vi "SEA_TORQUE_CONTROL_BENCHMARKING_TEST.vi"() -> ()   [LabVIEW 2019]
uses:
  <vilib>/FPGAPlugInAG/sbRIO-9627/niLvFpga_Open_sbRIO-9627.vi
  <vilib>/rvi/interface/common/dynamic/niFpgaDynamicAddResources.vi
  <vilib>/Utility/error.llb/Error Cluster From Error Code.vi
  <vilib>/rvi/errors/niLvFpgaAdjustHostInterfaceError.vi
  <vilib>/FPGAPlugInAG/Dynamic/niLvFpga_Close_Dynamic.vi
  <vilib>/rvi/interface/nirviOpenFPGA/nirviOpenFPGA.xnode
  FPGA Bitfiles/seafinalexperime_FPGATarget_SEALOWERLEVELCON_meT+vsors+U.lvbitx
  SEA_LOWER_LEVEL_CONTROL.vi
  <vilib>/rvi/interface/nirviReadWriteControl/nirviReadWriteControl.xnode
  <vilib>/rvi/interface/nirviCloseFPGA/nirviCloseFPGA.xnode
  NiFpgaLv.dll
  <vilib>/rvi/interface/Simulation/niFpgaSimulationCallBeginRW.vi
panel:
  out "Loop rate":u32
  in  "Position Reset":bool
  in  "Position Reset joint side":bool
  in  "KpGain":sgl
  out "Current":cluster{sgl, "Filtered Current(M2)":sgl}(graph)
  out "Torque":cluster{sgl, sgl}(graph)
  out "control_ip":sgl
  out "motor direction":bool
  in  "lower limit":sgl
  in  "upper limit":sgl
  in  "Kp":sgl
  in  "Amplitude":sgl
  in  "frequency":sgl
  in  "Current Offset":sgl
  in  "stop":bool
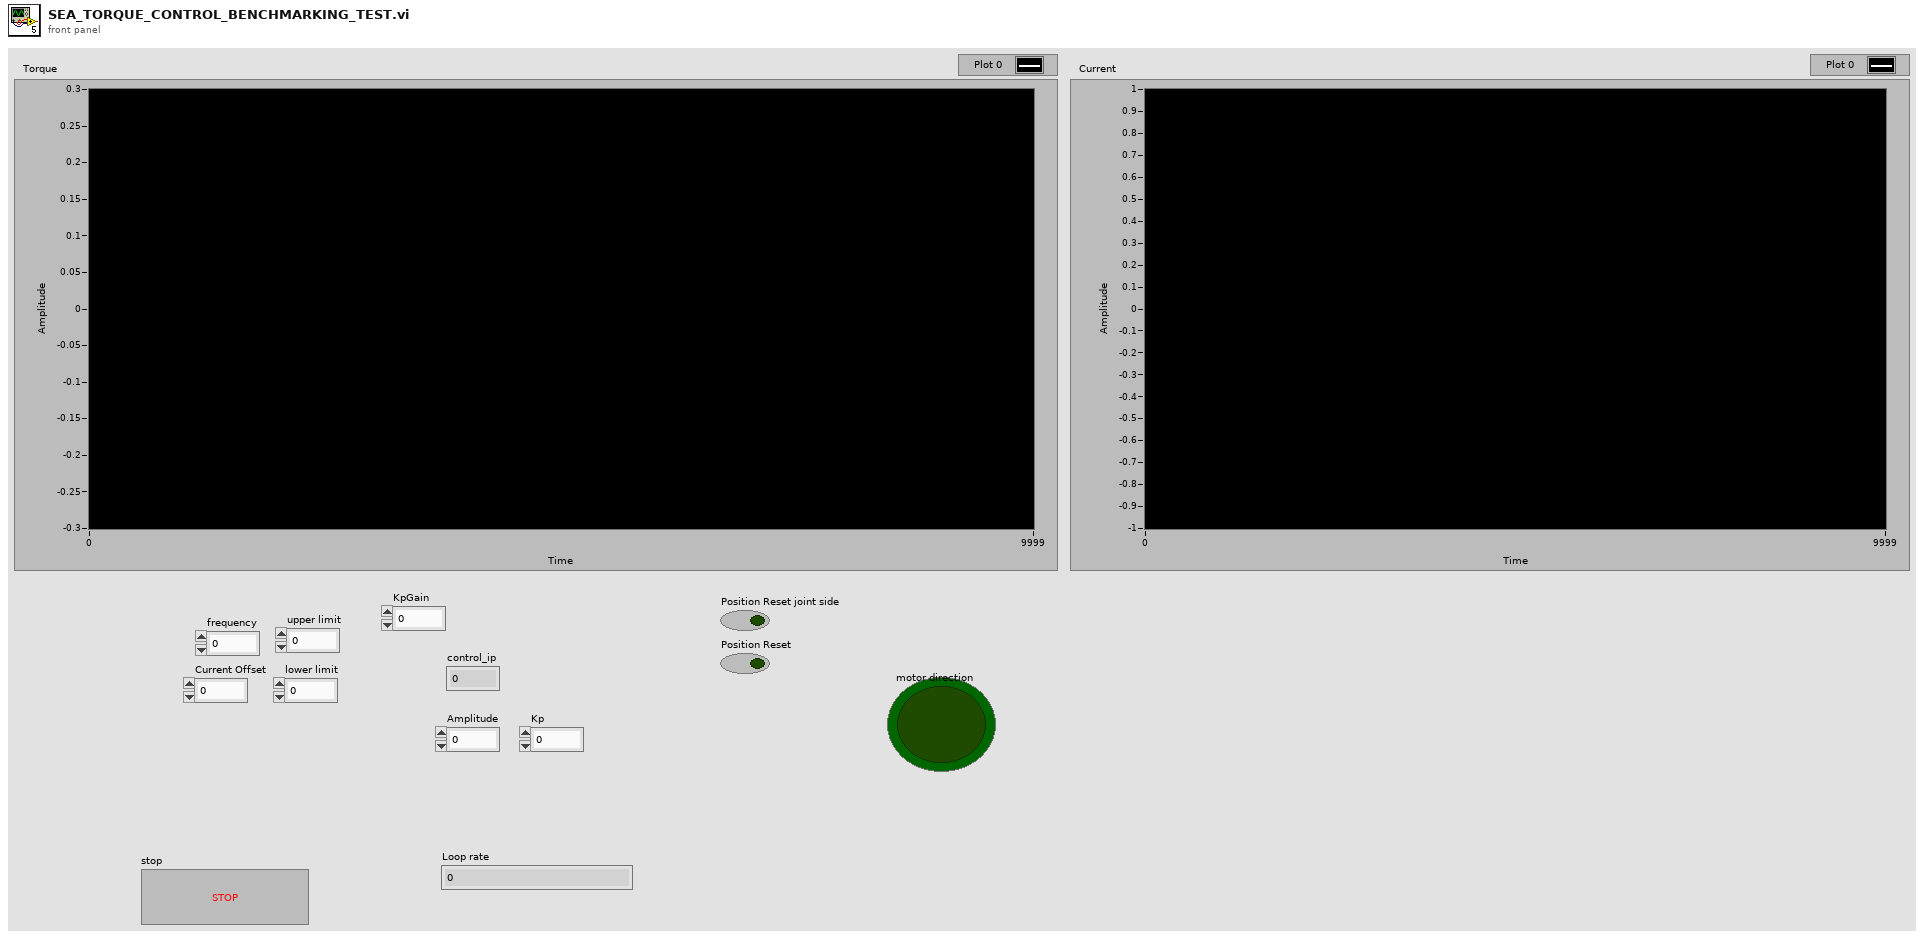
[diagram p1: front panel]
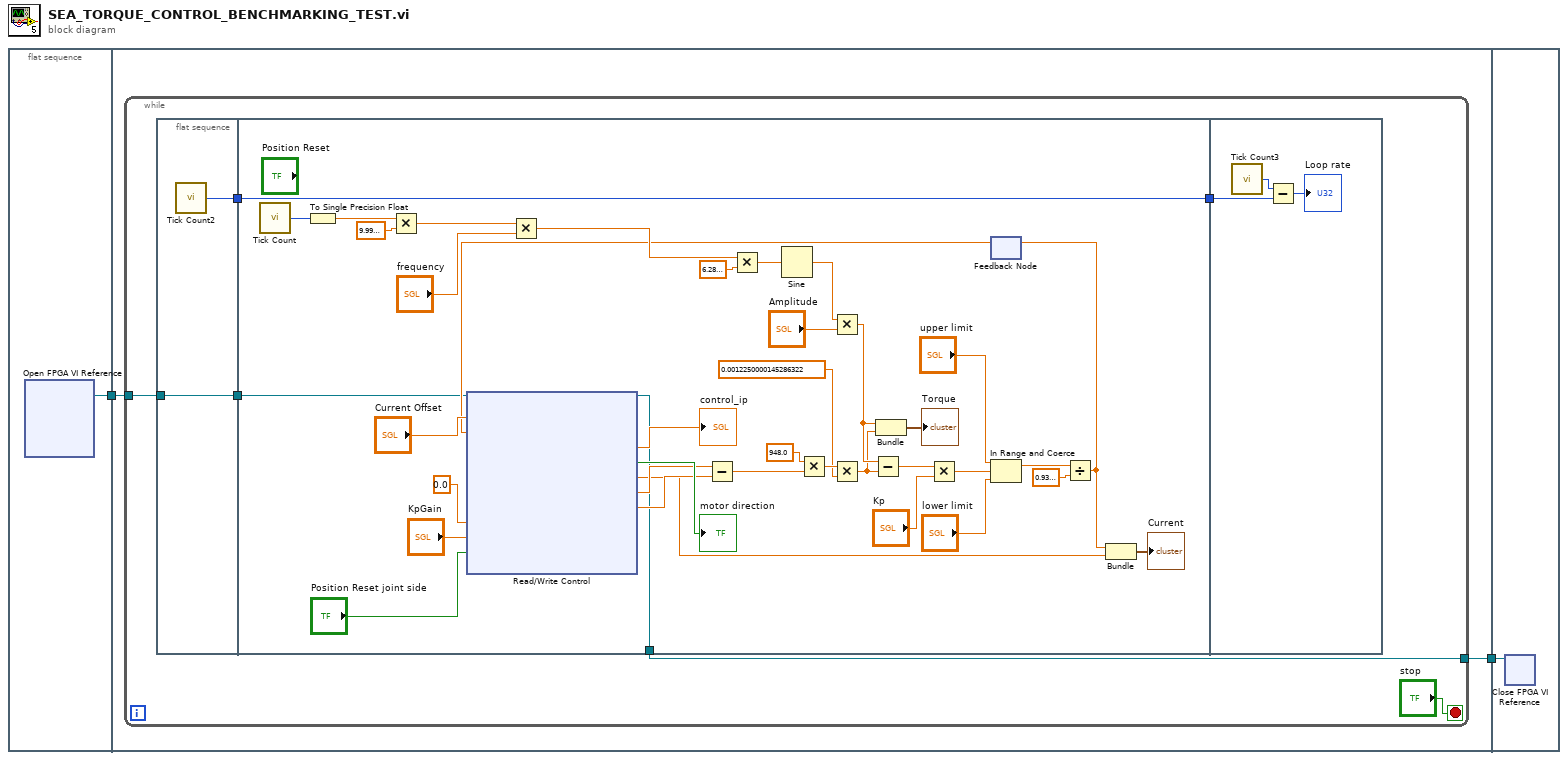
[diagram p0: block diagram]
diagram:
  n1 = flat-sequence {
    tunnel: [w3] -> w2
    tunnel: w2 -> [w5]
    tunnel: [w4] -> w1
    tunnel: w1 -> [w56]
    frame #0 {
      n2 = xnode "Open FPGA VI Reference"() -> ("FPGA VI Reference Out"=w3:refnum<k20>)  [unwired: 2 in, 1 out]
    }
    frame #1 {
      n3 = while {
        tunnel: w5 -> [w9]
        tunnel: [w8] -> w4
        stop <- "stop" stop-if-true
        n4 = flat-sequence {
          tunnel: [w13] -> w10
          tunnel: w9 -> [w13]
          tunnel: [w12] -> w7
          tunnel: w10 -> [w16]
          tunnel: [w15] -> w8
          tunnel: w7 -> [w14]
          tunnel: [w14] -> w6
          tunnel: w6 -> [w54]
          frame #0 {
            n5 = call "Tick Count2"() -> ("Tick Count(uSec)"=w12:u32)
          }
          frame #1 {
            n6 = call "Tick Count"() -> ("Tick Count(uSec)"=w26:u32)
            n7 = To Single Precision Float(number=w26) -> (single precision float=w25:sgl)
            n8 = Multiply(x=w25, y=sgl 1e-06) -> (x*y=w23:sgl)
            n9 = Multiply(x=w23, y="frequency") -> (x*y=w49:sgl)
            n10 = Multiply(x=w49, y=sgl 6.28) -> (x*y=w47:sgl)
            n11 = Sine(x=w47) -> (sin(x)=w46:sgl)
            n12 = Multiply(x=w46, y="Amplitude") -> (x*y=w34:sgl)
            n13 = feedback #1() -> (w35:sgl)  [unwired: 1 in]
            n14 = xnode "Read/Write Control"("FPGA VI Reference In"=w16, "Current Offset"="Current Offset", "reference"=w35, "Tracking zero offset"=sgl 0.0, "KpGain"="KpGain", "Position Reset joint side"="Position Reset joint side") -> ("FPGA VI Reference Out"=w15:refnum<k20>, "control_ip"=→"control_ip":sgl, "motor direction"=→"motor direction":bool, "Filtered Current(M2)"=w27:sgl, "Position(Radians) motor side"=w31:sgl, "Position(Radians) joint side"=w30:sgl)  [unwired: 2 in, 1 out]
            n15 = Subtract(x=w31, y=w30) -> (x-y=w51:sgl)
            n16 = Multiply(x=sgl 948.0, y=w51) -> (x*y=w50:sgl)
            n17 = Multiply(x=w50, y=sgl 0.001225) -> (x*y=w33:sgl)
            n18 = Subtract(x=w34, y=w33) -> (x-y=w44:sgl)
            n19 = Bundle(w34, w33) -> (→"Torque":cluster{sgl, sgl})  [unwired: 1 in]
            n20 = Multiply(x=w44, y="Kp") -> (x*y=w42:sgl)
            n21 = In Range and Coerce(upper limit="upper limit", x=w42, lower limit="lower limit") -> (coerced(x)=w39:sgl)  [unwired: 1 out]
            n22 = Divide(x=w39, y=sgl 0.94) -> (x/y=w17:sgl)
            n23 = feedback-in #1(w17) -> ()
            n24 = Bundle(w17, "Filtered Current(M2)"=w27) -> (→"Current":cluster{sgl, "Filtered Current(M2)":sgl})  [unwired: 1 in]
          }
          frame #2 {
            n25 = call "Tick Count3"() -> ("Tick Count(uSec)"=w55:u32)
            n26 = Subtract(x=w55, y=w54) -> (x-y=→"Loop rate":u32)
          }
        }
      }
    }
    frame #2 {
      n27 = xnode "Close FPGA VI Reference"("FPGA VI Reference In"=w56) -> ()  [unwired: 1 in, 1 out]
    }
  }
